vi "Bit Offset to Index.vi"(11 "bit offset":u64 format="%d bits") -> (2 "bit index":u8 format="%d bits", 3 "byte offset":u64 format="%d bytes")   [LabVIEW 2017, in "DSF Core.lvlib" / "Buffer Converter.lvclass"]
uses:
  Buffer Converter.lvclass
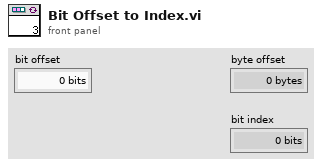
[diagram p1: front panel]
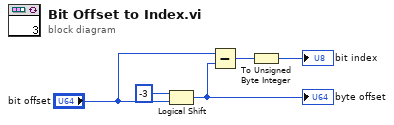
[diagram p0: block diagram]
diagram:
  n1 = Logical Shift(y=i16 -3, x="bit offset") -> (x << y=w4:u64)
  "byte offset" <- w4
  n2 = Subtract(x="bit offset", y=w4) -> (x-y=w2:u64)
  n3 = To Unsigned Byte Integer(number=w2) -> (unsigned 8bit integer=→"bit index":u8)
